vi "UpdatePump.vi"(0 "Pump_1AI_1DO_2DI in":refnum<class "ValveModbus.lvclass">, 2 "ARG U32":i32=100000, 5 "MB_ENGINE":refnum<class "MB_ENGINE.lvclass">, 9 "pressur":dbl format="%#_13g", 11 "error in (no error)":errorcluster) -> (4 "Pump_1AI_1DO_2DI out":refnum<class "ValveModbus.lvclass">, 6 "class data out":refnum<class "MB_ENGINE.lvclass">, 15 "error out":errorcluster)   [LabVIEW 2019, in "ValveModbus.lvclass"]
uses:
  ValveModbus.lvclass
  modbus engine custom/MB_ENGINE_class/MB_ENGINE.lvclass
  ValveModbus.lvclass/ValveModbus.ctl
  TypeDef/StateValveModbus.ctl
  modbus engine custom/MB_ENGINE_class/cmd enum.ctl
  da5bb0dd-82f2-4128-bc01-5250fa116678.vi
  389d00fe-f9cd-4760-9eba-55ad7c076291.vi
  24587cee-9224-44c2-8beb-c4414d14c72d.vi
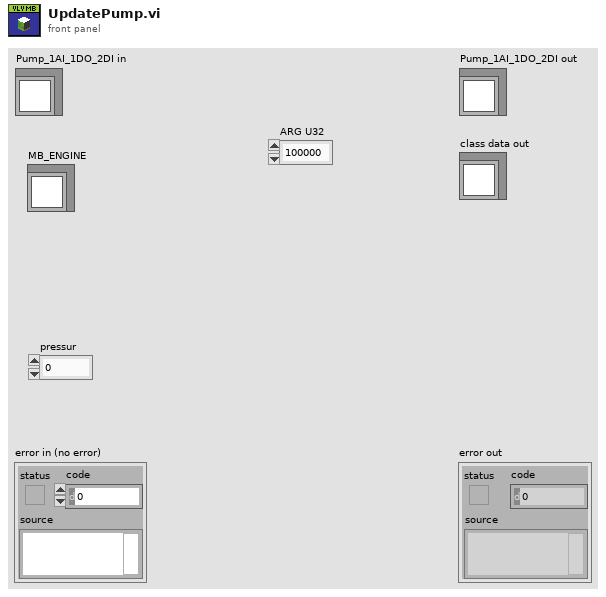
[diagram p1: front panel]
types:
  T1 = typedef "StateValveModbus.ctl" = enum16{"IDLE", "OPEN", "CLOSE", "OPENING", "CLOSING", "STOP"}
  T2 = typedef "MB_ENGINE.lvclass/Settings.ctl" = cluster{"ACC Steps Per Sec^2":u16, "DEC Steps Per Sec^2":u16, "Min Velosity Step Per Sec":u16, "Max Velosity Step Per Sec":u16, "MicroStep":u16}
  T3 = typedef "MB_ENGINE.lvclass/cmd enum.ctl" = u16
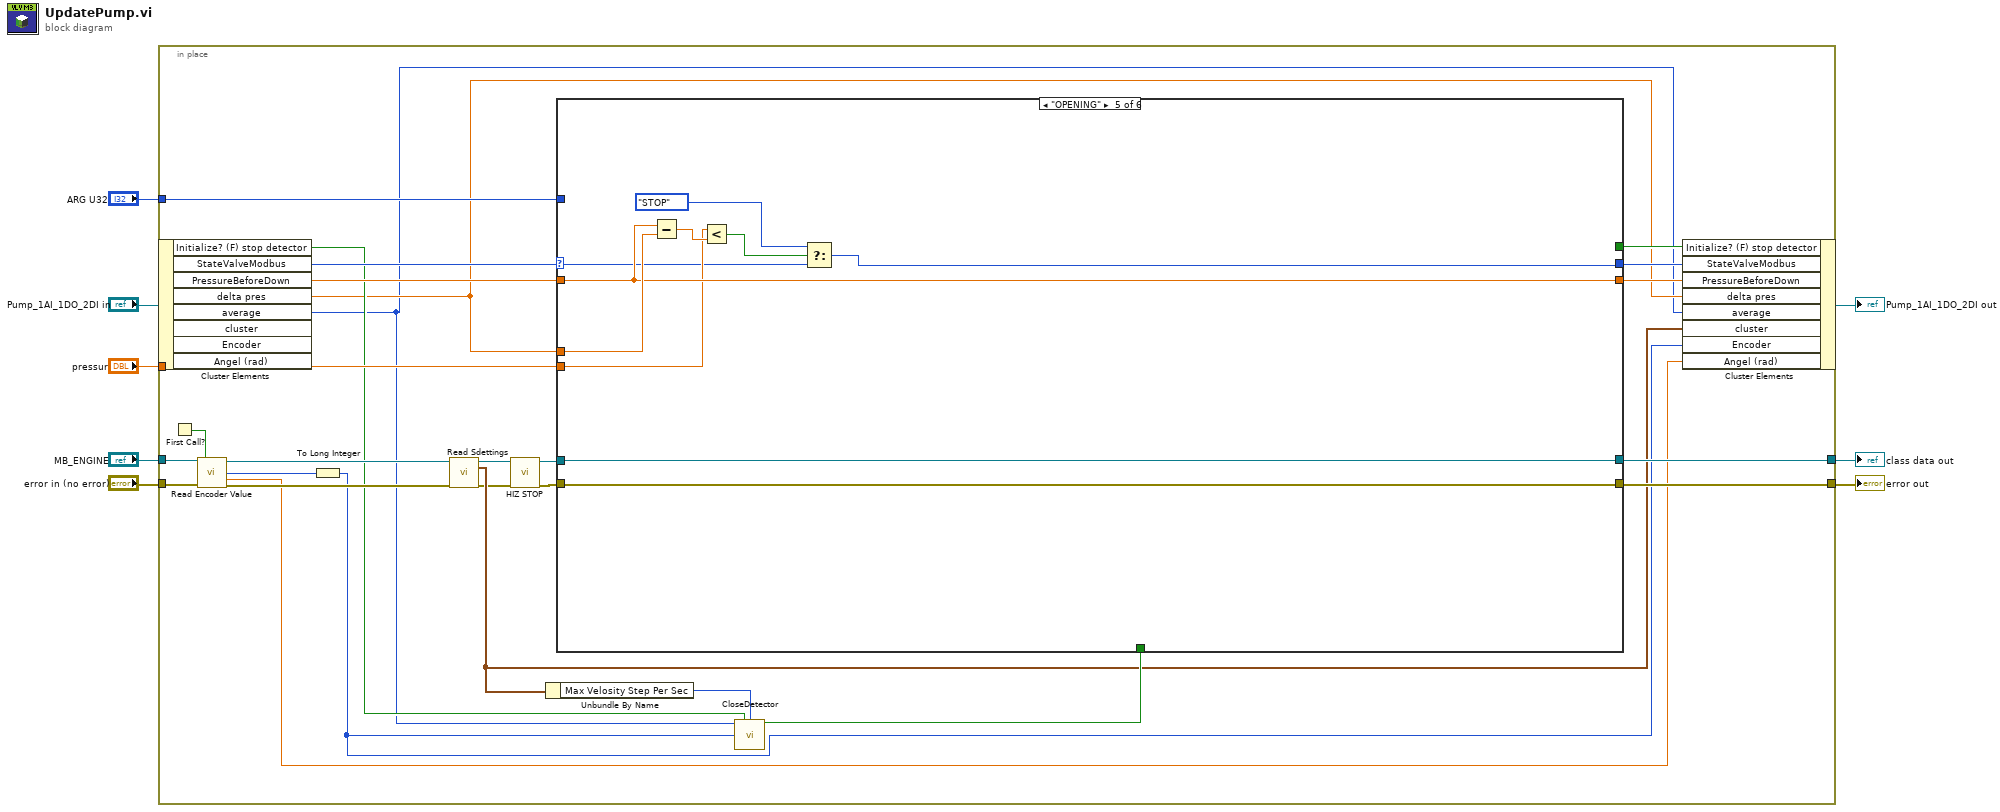
[diagram p0: block diagram]
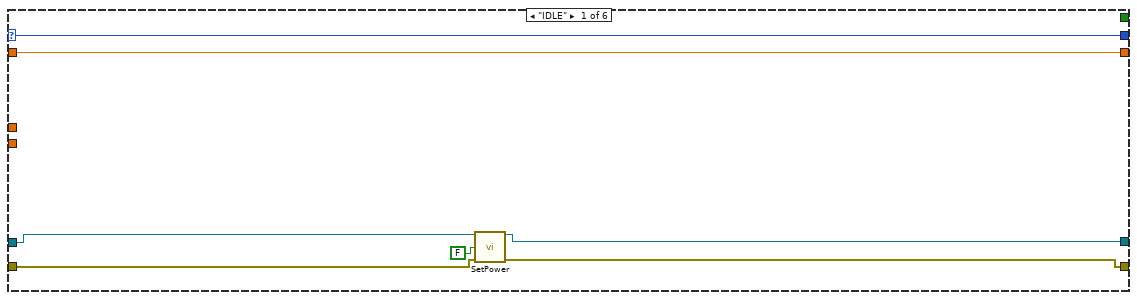
[diagram p2: hidden frame]
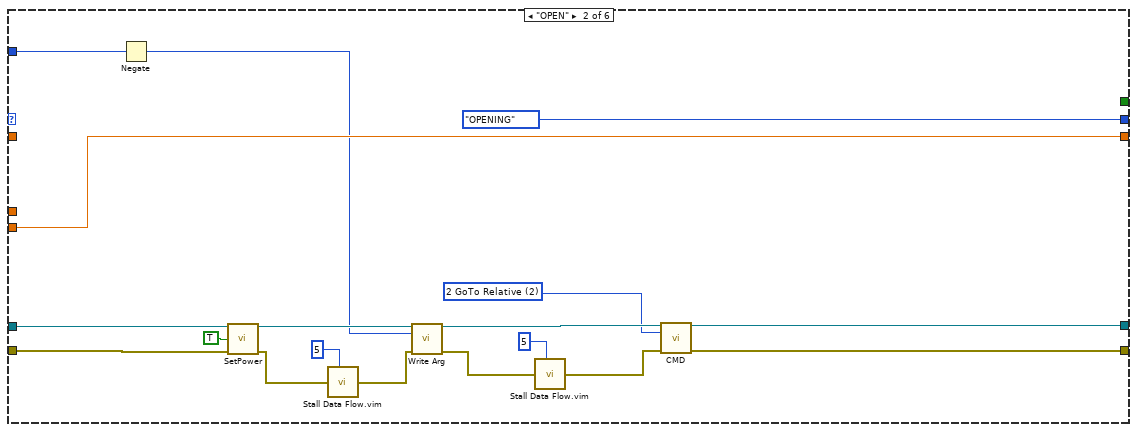
[diagram p3: hidden frame]
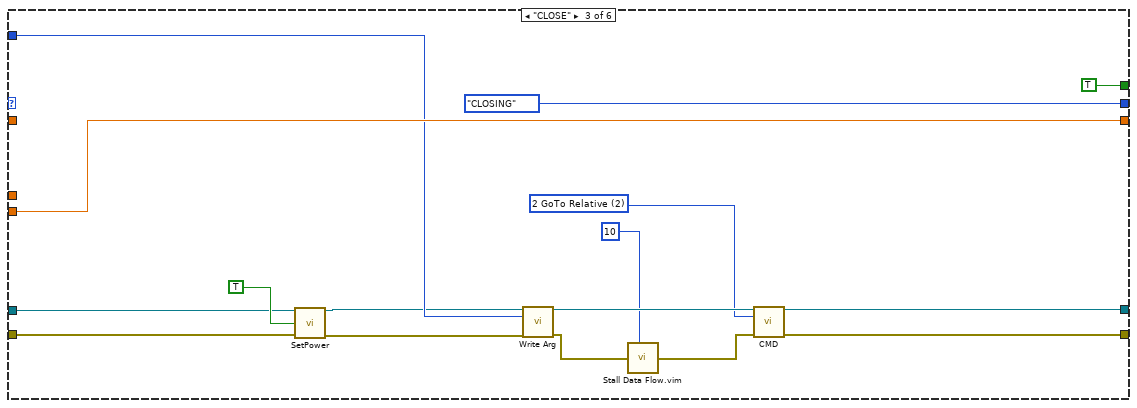
[diagram p4: hidden frame]
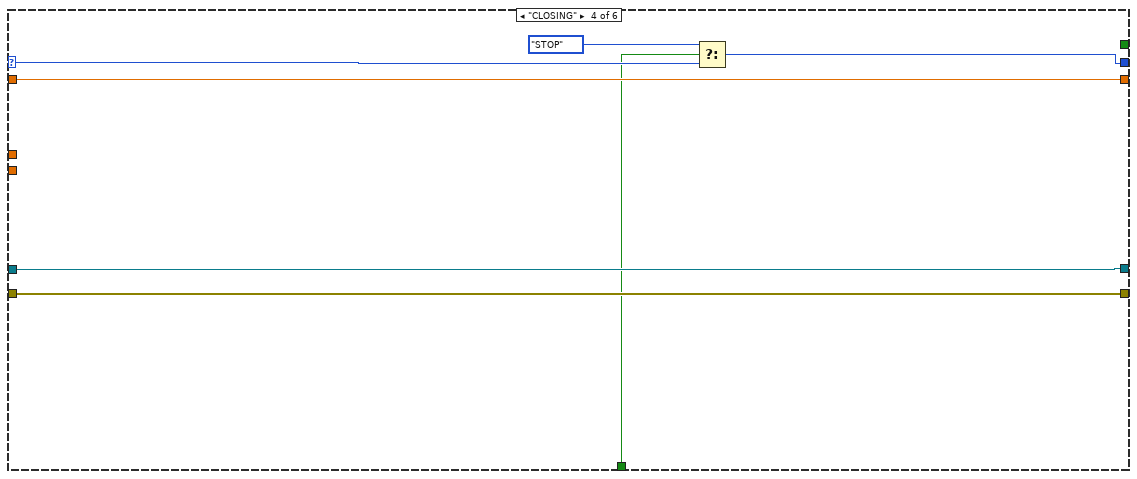
[diagram p5: hidden frame]
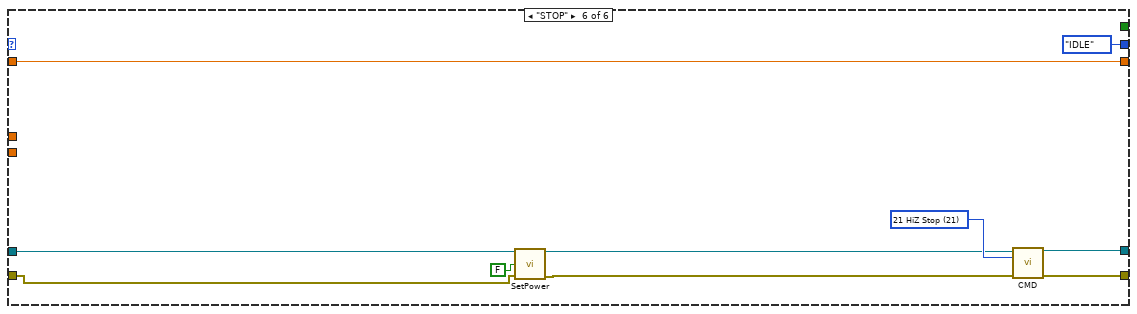
[diagram p6: hidden frame]
diagram:
  n1 = in-place {
    in-place-border: "error in (no error)" -> [w26]
    in-place-border: [w32] -> w5
    in-place-border: "MB_ENGINE" -> [w27]
    in-place-border: "pressur" -> [w30]
    in-place-border: "ARG U32" -> [w29]
    in-place-border: [w28] -> w1
    n2 = in-place-cluster #1("Pump_1AI_1DO_2DI in") -> ("Initialize? (F) stop detector"=w19:bool, "StateValveModbus"=w35:T1, "PressureBeforeDown"=w33:dbl, "delta pres"=w17:dbl, "average"=w16:i32)  [unwired: 3 out]
    n3 = First Call?() -> (First Call?: T/F=w24:bool)
    n4 = call-dynamic "Read Encoder Value.vi"("class data in"=w27, "init"=w24, "error in (no error)"=w26) -> ("class data out"=w23:refnum<class "MB_ENGINE.lvclass">, "Encoder"=w25:i32, "Angel (rad)"=w14:dbl, "error out"=w22:errorcluster)  [unwired: 8 in, 1 out]
    n5 = To Long Integer(number=w25) -> (32bit integer=w13:i32)
    n6 = call-dynamic "Read Sdettings.vi"("class data in"=w23, "error in (no error)"=w22) -> ("class data out"=w12:refnum<class "MB_ENGINE.lvclass">, "cluster"=w15:T2, "error out"=w11:errorcluster)  [unwired: 11 in]
    n7 = call-dynamic "HIZ STOP.vi"("class data in"=w12, "error in (no error)"=w11) -> ("class data out"=w9:refnum<class "MB_ENGINE.lvclass">, "error out"=w10:errorcluster)  [unwired: 12 in]
    n8 = Unbundle By Name(w15) -> ("Max Velosity Step Per Sec"=w21:u16)
    n9 = call "CloseDetector.vi"("Averaging Size"=w16, "Initialize? (F)"=w19, "MaxVelosity"=w21, "ENCODER"=w13) -> ("stop"=w18:bool)  [unwired: 11 in]
    n10 = case shown="\"OPENING\"" w35 {
      selector: w35 -> [w41 _ _ w80 w89 _]
      tunnel: [w42 w59 w76 w81 w92 w103] -> w34
      tunnel: w33 -> [w42 _ _ w81 w92 w103]
      tunnel: [w36 w55 w72 w82 w84 w101] -> w32
      tunnel: [w41 StateValveModbus."OPENING" ("StateValveModbus") StateValveModbus."CLOSING" ("StateValveModbus") w78 w87 StateValveModbus."IDLE" ("StateValveModbus")] -> w31
      tunnel: w30 -> [_ w59 w76 _ w90 _]
      tunnel: w29 -> [_ w60 w67 _ _ _]
      tunnel: [w37 w56 w73 w83 w85 w102] -> w28
      tunnel: w17 -> [_ _ _ _ w93 _]
      tunnel: w9 -> [w39 w50 w65 w83 w85 w97]
      tunnel: w10 -> [w38 w49 w64 w82 w84 w96]
      tunnel: [_ _ TRUE ("Initialize? (F) stop detector") _ _ _] -> w20
      tunnel: w18 -> [_ _ _ w79 _ _]
      frame "IDLE" {
        n11 = call-dynamic "SetPower.vi"("class data in"=w39, "On"=FALSE, "error in (no error)"=w38) -> ("class data out"=w37:refnum<class "MB_ENGINE.lvclass">, "error out"=w36:errorcluster)  [unwired: 11 in]
      }
      frame "OPEN" {
        w54 = T3 2 items=["0 Idle"=0, "1 GoTo Absolute Position"=1, "2 GoTo Relative"=2, "10 GoTo Home Position"=10, "11 Set Home Position"=11, "12 Set FindHome Mode"=12, "13 Reset FindHome Mode"=13, "14 Get FindHome State"=14, "20 Hard Stop"=20, "21 HiZ Stop"=21, "22 Soft Stop"=22, "30 Clear Fault"=30, "40 Encoder Set Home"=40, "70 Driver Init"=70] ("cmd to write")
        n12 = Negate(x=w60) -> (-x=w43:i32)
        n13 = call-dynamic "SetPower.vi"("class data in"=w50, "On"=TRUE, "error in (no error)"=w49) -> ("class data out"=w44:refnum<class "MB_ENGINE.lvclass">, "error out"=w46:errorcluster)  [unwired: 11 in]
        n14 = call "Stall Data Flow.vim"("value in"=w46, "milliseconds to wait"=u32 5) -> ("value out"=w45:errorcluster)  [unwired: 1 out]
        n15 = call-dynamic "Write Arg.vi"("class data in"=w44, "ARG U32"=w43, "error in (no error)"=w45) -> ("class data out"=w57:refnum<class "MB_ENGINE.lvclass">, "error out"=w53:errorcluster)  [unwired: 11 in]
        n16 = call "Stall Data Flow.vim"("value in"=w53, "milliseconds to wait"=u32 5) -> ("value out"=w51:errorcluster)  [unwired: 1 out]
        n17 = call-dynamic "CMD.vi"("class data in"=w57, "cmd to write"=w54, "error in (no error)"=w51) -> ("class data out"=w56:refnum<class "MB_ENGINE.lvclass">, "error out"=w55:errorcluster)  [unwired: 11 in]
      }
      frame "CLOSE" {
        w71 = T3 2 items=["0 Idle"=0, "1 GoTo Absolute Position"=1, "2 GoTo Relative"=2, "10 GoTo Home Position"=10, "11 Set Home Position"=11, "12 Set FindHome Mode"=12, "13 Reset FindHome Mode"=13, "14 Get FindHome State"=14, "20 Hard Stop"=20, "21 HiZ Stop"=21, "22 Soft Stop"=22, "30 Clear Fault"=30, "40 Encoder Set Home"=40, "70 Driver Init"=70] ("cmd to write")
        n18 = call-dynamic "SetPower.vi"("class data in"=w65, "On"=TRUE, "error in (no error)"=w64) -> ("class data out"=w62:refnum<class "MB_ENGINE.lvclass">, "error out"=w63:errorcluster)  [unwired: 11 in]
        n19 = call-dynamic "Write Arg.vi"("class data in"=w62, "ARG U32"=w67, "error in (no error)"=w63) -> ("class data out"=w74:refnum<class "MB_ENGINE.lvclass">, "error out"=w70:errorcluster)  [unwired: 11 in]
        n20 = call "Stall Data Flow.vim"("value in"=w70, "milliseconds to wait"=u32 10) -> ("value out"=w68:errorcluster)  [unwired: 1 out]
        n21 = call-dynamic "CMD.vi"("class data in"=w74, "cmd to write"=w71, "error in (no error)"=w68) -> ("class data out"=w73:refnum<class "MB_ENGINE.lvclass">, "error out"=w72:errorcluster)  [unwired: 11 in]
      }
      frame "CLOSING" {
        n22 = Select(t=StateValveModbus."STOP", s=w79, f=w80) -> (s? t:f=w78:T1)
      }
      frame "OPENING" {
        n23 = Subtract(x=w92, y=w93) -> (x-y=w91:dbl)
        n24 = Less?(x=w90, y=w91) -> (x < y?=w86:bool)
        n25 = Select(t=StateValveModbus."STOP", s=w86, f=w89) -> (s? t:f=w87:T1)
      }
      frame "STOP" {
        w100 = T3 21 items=["0 Idle"=0, "1 GoTo Absolute Position"=1, "2 GoTo Relative"=2, "10 GoTo Home Position"=10, "11 Set Home Position"=11, "12 Set FindHome Mode"=12, "13 Reset FindHome Mode"=13, "14 Get FindHome State"=14, "20 Hard Stop"=20, "21 HiZ Stop"=21, "22 Soft Stop"=22, "30 Clear Fault"=30, "40 Encoder Set Home"=40, "70 Driver Init"=70] ("cmd to write")
        n26 = call-dynamic "SetPower.vi"("class data in"=w97, "On"=FALSE, "error in (no error)"=w96) -> ("class data out"=w94:refnum<class "MB_ENGINE.lvclass">, "error out"=w95:errorcluster)  [unwired: 11 in]
        n27 = call-dynamic "CMD.vi"("class data in"=w94, "cmd to write"=w100, "error in (no error)"=w95) -> ("class data out"=w102:refnum<class "MB_ENGINE.lvclass">, "error out"=w101:errorcluster)  [unwired: 11 in]
      }
    }
    n28 = in-place-cluster #1("Initialize? (F) stop detector"=w20, "StateValveModbus"=w31, "PressureBeforeDown"=w34, "delta pres"=w17, "average"=w16, "cluster"=w15, "Encoder"=w13, "Angel (rad)"=w14) -> (→"Pump_1AI_1DO_2DI out":refnum<class "ValveModbus.lvclass">)
  }
  "error out" <- w5
  "class data out" <- w1
